vi "ButtonCanGrabberUp.vi"(11 "Buttons":bool[](array[boolean])) -> ()   [LabVIEW 2014]
uses:
  Utilities/CanGrabberSetpoint.vi
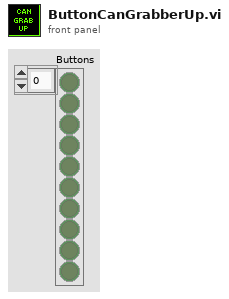
[diagram p1: front panel]
types:
  T1 = typedef "WPI_MotorControlDeviceRef.ctl" = cluster{"DeviceStatus":errorcluster, "Type":T2, "PWM":cluster{"Controller":T3, "PWM Channel":T4, "DeadBand":T5}, "CAN":cluster{"Device Number":u8, "Control Mode":T6, "Semaphore":T7, "Max Vout":dbl, "TalonSRX Control Mode":T8}, "Invert":bool, "TransformRef":T9, "InvTransformRef":T9}
  T2 = typedef "WPI_MotorControlType.ctl" = enum16{"PWM", "CAN", "CANTalonSRX"}
  T3 = typedef "FPGA_TypedefDigitalModule.ctl" = enum16{"Controller 1"}
  T4 = typedef "FPGA_DIOPWMChannel.ctl" = enum8{"PWM 0", "PWM 1", "PWM 2", "PWM 3", "PWM 4", "PWM 5", "PWM 6", "PWM 7", "PWM 8", "PWM 9", "PWM MXP 0", "PWM MXP 1", "PWM MXP 2", "PWM MXP 3", "PWM MXP 4", "PWM MXP 5", "PWM MXP 6", "PWM MXP 7", "PWM MXP 8", "PWM MXP 9", "Invalid"}
  T5 = typedef "WPI_PWMDeadband.ctl" = cluster{"Name":string, "maxPositivePwm":i32, "minPositivePwm":i32, "centerPwm":i32, "maxNegativePwm":i32, "minNegativePwm":i32, "angularRange":u16}
  T6 = typedef "WPI_CANJaguar_ControlMode.ctl" = enum8{"Percent VBus", "Current", "Speed", "Position", "Voltage"}
  T7 = typedef "Semaphore RefNum" = refnum<k1>
  T8 = typedef "WPI_CANTalonSRX_APIControlMode.ctl" = enum8{"Percent VBus", "Speed", "Position", "Slave", "Unchanged / Invalid"}
  T9 = typedef "WPI_PWMTransform_ConPane.ctl" = refnum<vi>
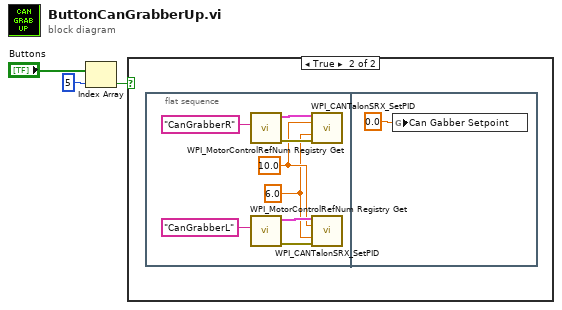
[diagram p0: block diagram]
diagram:
  n1 = Index Array(array="Buttons", index=5) -> (element=w2:bool)
  n2 = case shown="True" w2 {
    frame False {
    }
    frame True {
      n3 = flat-sequence {
        frame #0 {
          w4 = 6.0 ("D")
          w5 = 10.0 ("P")
          n4 = call <vilib>:"WPI_MotorControlRefNum Registry Get.vi"("refnum name"="CanGrabberR") -> ("error out"=w7:errorcluster, "MotorControlDevRef"=w6:T1)  [unwired: 9 in]
          n5 = call <vilib>:"WPI_MotorControlRefNum Registry Get.vi"("refnum name"="CanGrabberL") -> ("error out"=w8:errorcluster, "MotorControlDevRef"=w9:T1)  [unwired: 9 in]
          n6 = call <vilib>:"WPI_CANTalonSRX_SetPID.vi"("CAN Talon SRX Ref"=w6, "P"=w5, "D"=w4, "error in (no error)"=w7) -> ()  [unwired: 10 in, 2 out]
          n7 = call <vilib>:"WPI_CANTalonSRX_SetPID.vi"("CAN Talon SRX Ref"=w9, "P"=w5, "D"=w4, "error in (no error)"=w8) -> ()  [unwired: 10 in, 2 out]
        }
        frame #1 {
          n8 = global write "CanGrabberSetpoint.vi" "Can Gabber Setpoint"(0.0 ("Output")) -> ()
        }
      }
    }
  }
